vi "Unregister.vi"(0 "WebFrontPanel":refnum<class "WebFrontPanel.lvclass">, 5 "error in (no error)":errorcluster) -> (19 "error out":errorcluster)   [LabVIEW 2014, in "FrontPanelPublisher.lvlib" / "FrontPanelManager.lvclass"]
doc: "Unregister a WebFrontPanel"
uses:
  FrontPanelManager.lvclass
  WebFrontPanel_class/WebFrontPanel.lvclass
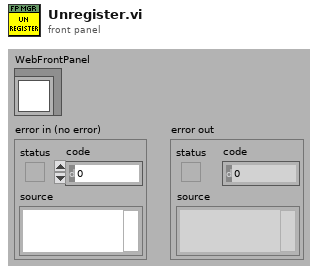
[diagram p1: front panel]
types:
  T1 = typedef "FrontPanelPublisher.lvlib/FrontPanelManager.lvclass/ObjectAttributes.ctl" = cluster{"WebFrontPanels":refnum<class "WebFrontPanel.lvclass">[], "WFP Names":string[], "Root folder":path, "Websocket Info":T2}
  T2 = typedef "FrontPanelPublisher.lvlib/FrontPanelManager.lvclass/WebsocketInfo.ctl" = cluster{"Hostname":string, "Port":u16}
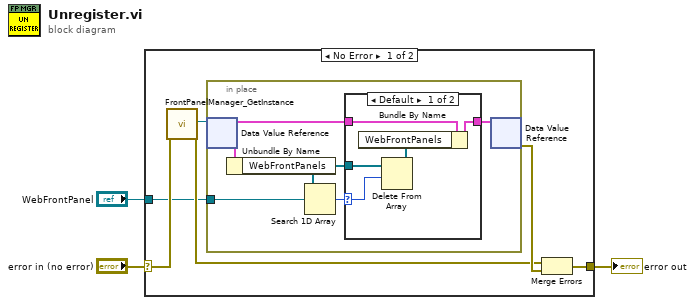
[diagram p0: block diagram]
diagram:
  n1 = case shown="No Error" "error in (no error)" {
    selector: "error in (no error)" -> [w7 w21]
    tunnel: [w8 w21] -> w2
    tunnel: "WebFrontPanel" -> [w4 _]
    frame No Error {
      n2 = call "FrontPanelManager_GetInstance.vi"("error in (no error)"=w7) -> ("DVRRefOut"=w5:refnum<data-value>, "error out"=w6:errorcluster)  [unwired: 14 in, 3 out]
      n3 = in-place {
        in-place-border: w4 -> [w10]
        n4 = in-place-dvr #1(w5) -> (w13:T1)  [unwired: 1 out]
        n5 = Unbundle By Name(w13) -> ("WebFrontPanels"=w11:refnum<class "WebFrontPanel.lvclass">[])
        n6 = Search 1D Array(1D array=w11, element=w10) -> (index of element=w14:i32)  [unwired: 1 in]
        n7 = case shown="Default" w14 {
          selector: w14 -> [w15 _]
          tunnel: [w18 w20] -> w12
          tunnel: w13 -> [w19 w20]
          tunnel: w11 -> [w17 _]
          frame Default {
            n8 = Delete From Array(array=w17, length=w15) -> (deleted portion=w16:refnum<class "WebFrontPanel.lvclass">[])  [unwired: 1 in, 1 out]
            n9 = Bundle By Name(cluster=w19, "WebFrontPanels"=w16) -> (w18:T1)
          }
          frame -1 {
          }
        }
        n10 = in-place-dvr #1(w12) -> (w9:errorcluster)  [unwired: 1 out]
      }
      n11 = Merge Errors(w6, w9) -> (w8:errorcluster)
    }
    frame Error {
    }
  }
  "error out" <- w2
